vi "Is Synced to Scan.vi"(8 "error in":errorcluster, 11 "Item Ref in":T1 format="%.0x") -> (0 "error out":errorcluster, 1 "Engine Rate":dbl, 2 "Sync to Scan?":bool, 3 "Item Ref out":T1 format="%.0x")   [LabVIEW 2016, in "Scan Engine Custom Device.lvlib"]
uses:
  Scan Engine Custom Device.lvlib
  <vilib>/NI Veristand/Custom Device API/Custom Device Item Ref.ctl
  NationalInstruments.VeriStand.SystemStorage
  <vilib>/NI Veristand/Custom Device Tools/Custom Device Utility Library/Custom Device Utility Library.lvlib
  <vilib>/NI Veristand/Custom Device API/Custom Device API.lvlib
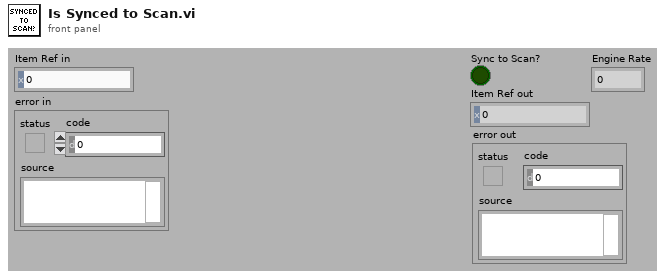
[diagram p1: front panel]
types:
  T1 = typedef "Custom Device API.lvlib/Custom Device Item Ref.ctl" = u64
  T2 = typedef "Custom Device API.lvlib/Custom Device Pointer.ctl" = refnum<k24>
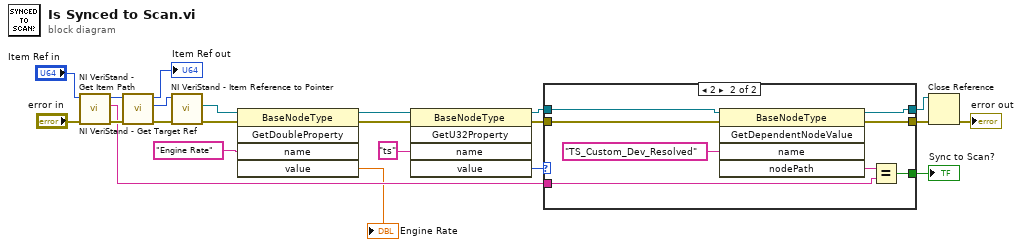
[diagram p0: block diagram]
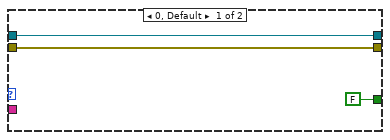
[diagram p2: hidden frame]
diagram:
  n1 = call <vilib>:"NI VeriStand - Get Item Path.vi"("error in (no error)"="error in", "Item Ref in"="Item Ref in") -> ("error out"=w14:errorcluster, "Path"=w11:string, "Item Ref out"=w15:T1)  [unwired: 6 in, 1 out]
  n2 = call <vilib>:"NI VeriStand - Get Target Ref.vi"("error in"=w14, "Item Ref in"=w15) -> ("error out"=w19:errorcluster, "Target Ref"=w7:T1, "Item Ref out"=→"Item Ref out":T1)  [unwired: 6 in, 1 out]
  n3 = call <vilib>:"NI VeriStand - Item Reference to Pointer.vi"("error in (no error)"=w19, "Item Ref in"=w7) -> ("error out"=w3:errorcluster, "Node Pointer"=w4:T2)  [unwired: 6 in, 2 out]
  n4 = invoke class="BaseNodeType" method="GetDoubleProperty"(reference=w4, error in=w3, "name"="Engine Rate") -> (reference out=w5:T2, error out=w6:errorcluster, "value"=→"Engine Rate":dbl)  [unwired: 2 in, 2 out]
  n5 = invoke class="BaseNodeType" method="GetU32Property"(reference=w5, error in=w6, "name"="ts") -> (reference out=w22:T2, error out=w21:errorcluster, "value"=w18:u32)  [unwired: 2 in, 2 out]
  n6 = case shown="2" w18 {
    tunnel: w22 -> [w24 w33]
    tunnel: w21 -> [w23 w32]
    tunnel: [FALSE w28] -> w17
    tunnel: w11 -> [_ w29]
    tunnel: [w24 w27] -> w10
    tunnel: [w23 w26] -> w9
    frame 0, Default {
    }
    frame 2 {
      n7 = invoke class="BaseNodeType" method="GetDependentNodeValue"(reference=w33, error in=w32, "name"="TS_Custom_Dev_Resolved") -> (reference out=w27:T2, error out=w26:errorcluster, "nodePath"=w30:string)  [unwired: 2 in, 2 out]
      n8 = Equal?(x=w30, y=w29) -> (x = y?=w28:bool)
    }
  }
  "Sync to Scan?" <- w17
  n9 = Close Reference(reference=w10, error in (no error)=w9) -> (error out=→"error out":errorcluster)
